vi "LabView360-6-Global-1.vi"() -> ()   [LabVIEW 2017]
uses:
  LabView360-6-Global.vi
panel:
  out "波形图表":dbl(graph)
  in  "停止":bool
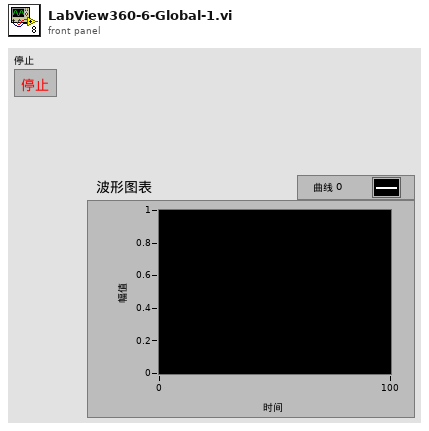
[diagram p1: front panel]
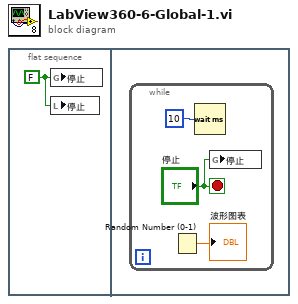
[diagram p0: block diagram]
diagram:
  n1 = flat-sequence {
    frame #0 {
      w1 = FALSE ("停止")
      n2 = global write "LabView360-6-Global.vi" "停止"(w1) -> ()
      n3 = local write "停止"(w1) -> ()
    }
    frame #1 {
      n4 = while {
        stop <- "停止" stop-if-true
        n5 = Random Number (0-1)() -> (number: 0 to 1=→"波形图表":dbl)
        n6 = Wait (ms)(milliseconds to wait=u32 10 ("等待时间（毫秒）")) -> ()  [unwired: 1 out]
        n7 = global write "LabView360-6-Global.vi" "停止"("停止") -> ()
      }
    }
  }
